vi "Open URL in Default Browser.vi"   [LabVIEW 2015]
doc: "Displays a URL or HTML file in the default Web browser. If the URL or path you wire to this VI contains a space character, the VI encodes the space as %20 before displaying the URL or HTML file in the Web browser. Wire data to the <B>URL</B> input to determine the polymorphic instance to use or manually select the instance."
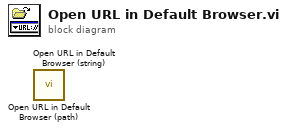
[diagram p0: block diagram]
diagram:
  n1 = call "Open URL in Default Browser (path).vi"() -> ()  [unwired: 6 in, 2 out]
  n2 = call "Open URL in Default Browser (string).vi"() -> ()  [unwired: 6 in, 2 out]
